vi "strings to line.vi"(11 "strings":string[](array[string])) -> (3 "line":T1)   [LabVIEW 2015, in "io editor node.lvclass"]
uses:
  io editor node.lvclass
  table line.ctl
  <vilib>/NI/Tag Bus Module Framework/channel/TBM channel.lvclass
  <vilib>/NI/Tag Bus/tag/Data Type.ctl
  permissions.ctl
  fpga channel/fpga channel.lvclass
  fifo channel/fifo channel.lvclass
  fifo channel/fifo channel.lvclass/fifo channel.ctl
  <vilib>/NI/Tag Bus/tag/tag descriptor.lvclass/tag descriptor.ctl
  <vilib>/NI/Tag Bus Module Framework/channel/TBM channel.lvclass/TBM channel.ctl
  <vilib>/NI/Tag Bus/tag/write tag name.vi
  <vilib>/NI/Tag Bus Module Framework/channel/Write channel classification.vi
  <vilib>/NI/Tag Bus/tag/write data type.vi
  <vilib>/NI/Tag Bus/tag/tag descriptor.lvclass
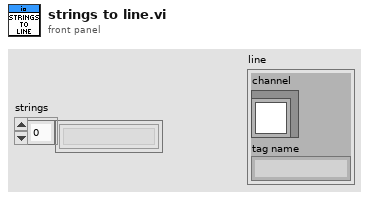
[diagram p1: front panel]
types:
  T1 = typedef "io editor node.lvclass/table line.ctl" = cluster{"channel":refnum<class "TBM channel.lvclass">, "tag name":string}
  T2 = typedef "io editor node.lvclass/permissions.ctl" = enum32{"Read from Indicator", "Write to Control"}
  T3 = typedef "tag bus.lvlib/tag descriptor.lvclass/Data Type.ctl" = enum16{"Double", "Single", "I64", "I32", "I16", "I8", "U64", "U32", "U16", "U8", "Boolean", "String", "Array of Double", "Array of Single", "Array of I64", "Array of I32", "Array of I16", "Array of I8", "Array of U64", "Array of U32", "Array of U16", "Array of U8", "Array of Boolean", "Array of String"}
  T4 = typedef "TBM channel.lvclass/channel classification.ctl" = enum16{"input data", "output data", "processing parameter", "processing result"}
  T5 = typedef "fifo channel.lvclass/fifo channel settings.ctl" = cluster{"Timeout":string, "Reset":string, "Averages":i32, "Samples":u32, "Channels":i32, "Fifo size":u32}
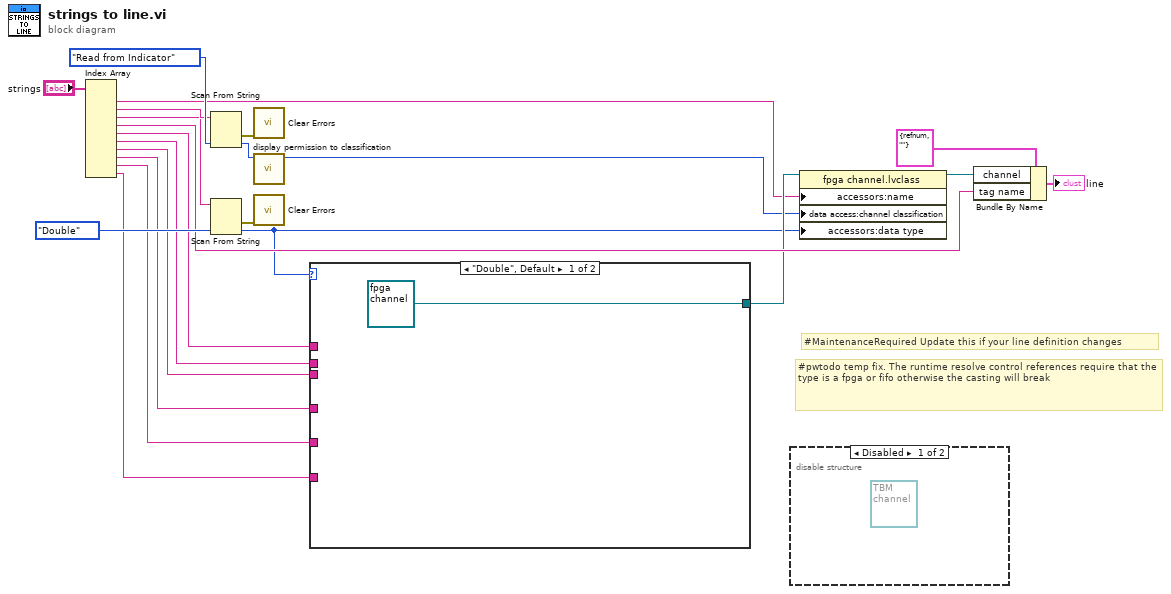
[diagram p0: block diagram]
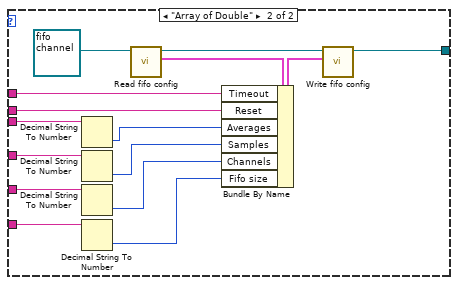
[diagram p3: hidden frame]
diagram:
  # "#pwtodo temp fix. The runtime resolve control references require that the type is a fpga or fifo otherwise the casting will break"
  # "#MaintenanceRequired Update this if your line definition changes"
  n1 = Index Array(array="strings") -> (element #1=w8:string, element #2=w15:string, element #3=w13:string, element #4=w12:string, element #5=w6:string, element #6=w5:string, element #7=w4:string, element #8=w3:string, element #9=w2:string, element #10=w1:string)  [unwired: 10 in]
  n2 = Scan From String(input string=w15, default 1=permissions."Read from Indicator" ("direction")) -> (error out=w17:errorcluster, output 1=w14:T2)  [unwired: 3 in, 2 out]
  n3 = Scan From String(input string=w13, default 1=Data_Type."Double" ("data type")) -> (error out=w19:errorcluster, output 1=w7:T3)  [unwired: 3 in, 2 out]
  n4 = call <vilib>:"Clear Errors.vi"("error in (no error)"=w17) -> ()  [unwired: 5 in, 2 out]
  n5 = call "display permission to classification.vi"("display permissions"=w14) -> ("channel classification"=w9:T4)  [unwired: 10 in]
  n6 = call <vilib>:"Clear Errors.vi"("error in (no error)"=w19) -> ()  [unwired: 5 in, 2 out]
  n7 = case shown="\"Double\", Default" w7 {
    tunnel: [refnum<class "fpga channel.lvclass"> refnum ("fpga channel.lvclass") w36] -> w11
    tunnel: w6 -> [_ w33]
    tunnel: w5 -> [_ w32]
    tunnel: w4 -> [_ w31]
    tunnel: w3 -> [_ w29]
    tunnel: w2 -> [_ w27]
    tunnel: w1 -> [_ w25]
    frame "Double", Default {
    }
    frame "Array of Double" {
      n8 = Decimal String To Number(string=w31) -> (number=w30:i32)  [unwired: 2 in, 1 out]
      n9 = Decimal String To Number(string=w29) -> (number=w28:i32)  [unwired: 2 in, 1 out]
      n10 = Decimal String To Number(string=w27) -> (number=w26:i32)  [unwired: 2 in, 1 out]
      n11 = Decimal String To Number(string=w25) -> (number=w24:i32)  [unwired: 2 in, 1 out]
      n12 = call "Read fifo config.vi"("fifo channel in"=refnum<class "fifo channel.lvclass"> refnum ("fifo channel.lvclass")) -> ("fifo config"=w35:T5, "fifo channel out"=w37:refnum<class "fifo channel.lvclass">)  [unwired: 8 in, 1 out]
      n13 = Bundle By Name(cluster=w35, "Timeout"=w33, "Reset"=w32, "Averages"=w30, "Samples"=w28, "Channels"=w26, "Fifo size"=w24) -> (w34:T5)
      n14 = call "Write fifo config.vi"("fifo config"=w34, "fifo channel in"=w37) -> ("fifo channel out"=w36:refnum<class "fifo channel.lvclass">)  [unwired: 8 in, 1 out]
    }
  }
  n15 = disable-structure shown="Disabled" {
    frame Disabled {
      (unwired) refnum<class "TBM channel.lvclass"> refnum ("channel")
    }
    frame Enabled {
    }
  }
  n16 = property class="fpga channel.lvclass"(reference=w11, "accessors:name"=w8, "data access:channel classification"=w9, "accessors:data type"=w7) -> (reference out=w10:refnum<class "fpga channel.lvclass">)  [unwired: 1 in, 1 out]
  n17 = Bundle By Name(cluster=T1 {"channel"=refnum, "tag name"=""} ("line"), "channel"=w10, "tag name"=w12) -> (→"line":T1)
